vi "음료자판기.vi"() -> ()   [LabVIEW 2014]
uses:
  <vilib>/Utility/miscctls.llb/LVOutOfRangeActionTypeDef.ctl
panel:
  in  "음료선택":u8(knob) max=2 step=1 scale=0.0..2.0
  in  "정지":bool
  in  "구매":bool
  in  "음료수량 초기값":cluster{"콜라":u8, "사이다":u8, "생수":u8}={"콜라"=10, "사이다"=10, "생수"=10}
  out "생수":u8
  out "사이다":u8
  out "콜라":u8
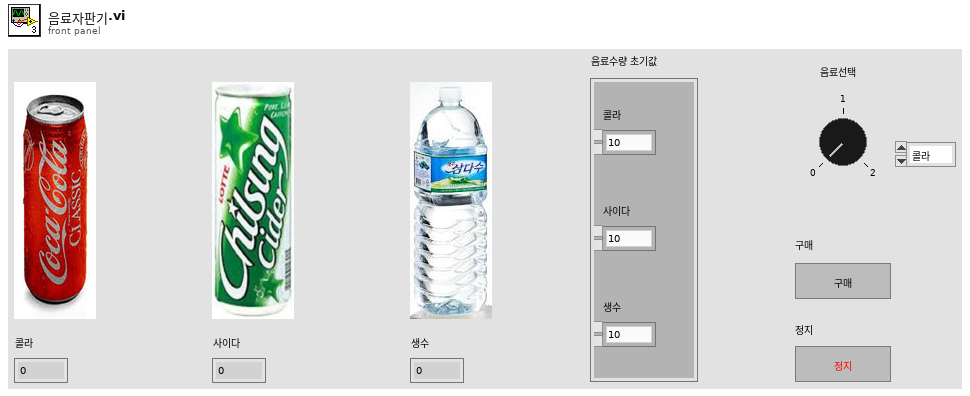
[diagram p1: front panel]
types:
  T1 = typedef "음료.ctl" = enum16{"Idle", "초기화", "정지", "음료확인", "구매"}
  T2 = typedef "LVOutOfRangeActionTypeDef.ctl" = cluster{"Out of Range Action Minimum":u8, "Out of Range Action Maximum":u8, "Out of Range Action Increment":u8}
  T3 = enum8{"Enabled", "Disabled", "Disabled and Grayed Out"}
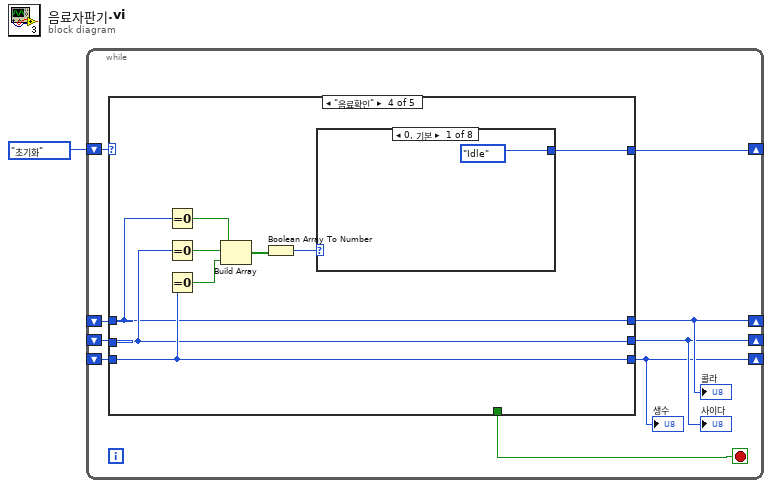
[diagram p0: block diagram]
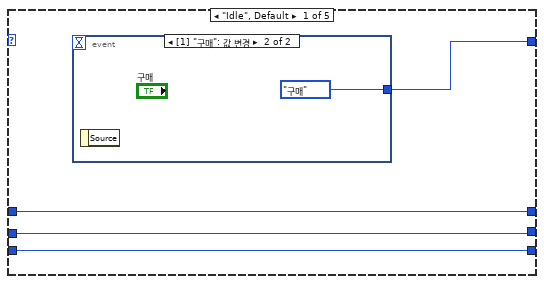
[diagram p2: hidden frame]
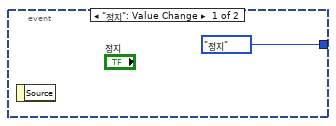
[diagram p3: hidden frame]
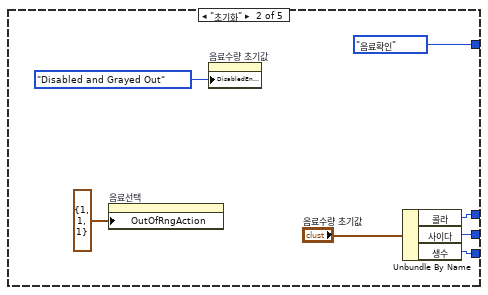
[diagram p4: hidden frame]
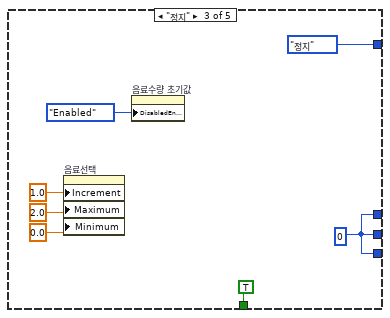
[diagram p5: hidden frame]
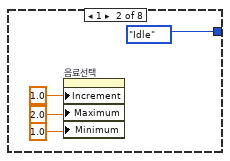
[diagram p6: hidden frame]
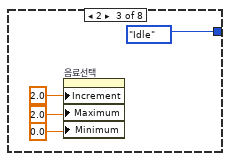
[diagram p7: hidden frame]
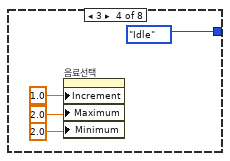
[diagram p8: hidden frame]
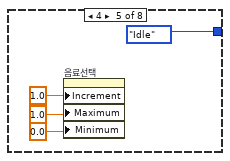
[diagram p9: hidden frame]
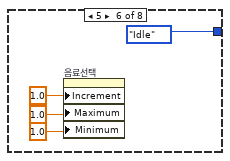
[diagram p10: hidden frame]
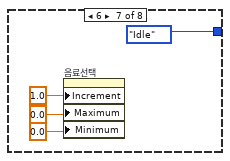
[diagram p11: hidden frame]
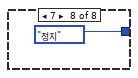
[diagram p12: hidden frame]
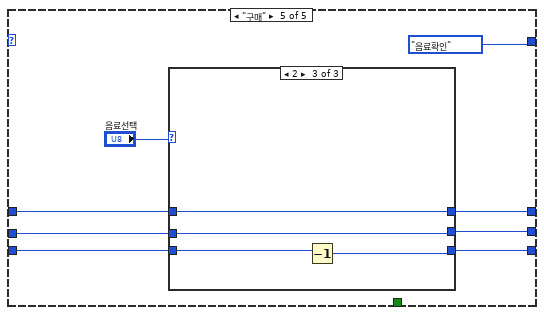
[diagram p13: hidden frame]
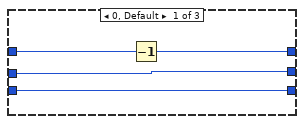
[diagram p14: hidden frame]
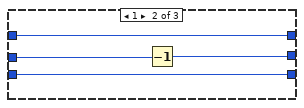
[diagram p15: hidden frame]
diagram:
  n1 = while {
    shift-right: [w9] -> _
    shift-left: 음료."초기화" ("열거형") -> [w10]
    shift-right: [w4] -> _
    shift-left: _ -> [w8]
    shift-right: [w3] -> _
    shift-left: _ -> [w7]
    shift-right: [w2] -> _
    shift-left: _ -> [w6]
    stop <- w5 stop-if-true
    n2 = case shown="\"음료확인\"" w10 {
      tunnel: [w14 음료."음료확인" ("열거형") 음료."정지" ("열거형") w31 음료."음료확인" ("열거형")] -> w9
      tunnel: w8 -> [w13 _ _ w37 w72]
      tunnel: w7 -> [w12 _ _ w38 w69]
      tunnel: w6 -> [w11 _ _ w39 w67]
      tunnel: [w13 w21 w24 w37 w71] -> w4
      tunnel: [w12 w20 w24 w38 w70] -> w3
      tunnel: [w11 w19 w24 w39 w68] -> w2
      tunnel: [_ _ TRUE _ _] -> w5
      frame "Idle", Default {
        n3 = event shown="[1] \"구매\": 값 변경" {
          selector: _ -> [_ _]
          dyn-events: _ -> [_ _]
          timeout: _ -> [_ _]
          tunnel: [음료."정지" ("열거형") 음료."구매" ("열거형")] -> w14
          event "정지": Value Change {
            n4 = event-data() -> ()  [unwired: 1 in, 1 out]
          }
          event "구매": Value Change {
            n5 = event-data() -> ()  [unwired: 1 in, 1 out]
          }
        }
      }
      frame "초기화" {
        n6 = property on="음료선택" class="Knob (엄격한)"("OutOfRngAction"=T2 {"Out of Range Action Minimum"=1, "Out of Range Action Maximum"=1, "Out of Range Action Increment"=1} ("리미트 밖의 값에 응답")) -> ()  [unwired: 2 in, 2 out]
        n7 = property on="음료수량 초기값" class="Clust (엄격한)"("DisabledEnum"=T3."Disabled and Grayed Out" ("비활성화")) -> ()  [unwired: 2 in, 2 out]
        n8 = Unbundle By Name("음료수량 초기값") -> ("콜라"=w21:u8, "사이다"=w20:u8, "생수"=w19:u8)
      }
      frame "정지" {
        w24 = 0
        n9 = property on="음료선택" class="Knob (엄격한)"("Increment"=1.0 ("데이터 입력 제한:증가"), "Maximum"=2.0 ("데이터 입력 제한:최대"), "Minimum"=0.0 ("데이터 입력 제한:최소")) -> ()  [unwired: 2 in, 2 out]
        n10 = property on="음료수량 초기값" class="Clust (엄격한)"("DisabledEnum"=T3."Enabled" ("비활성화")) -> ()  [unwired: 2 in, 2 out]
      }
      frame "음료확인" {
        n11 = Equal To 0?(x=w37) -> (x = 0?=w36:bool)
        n12 = Equal To 0?(x=w38) -> (x = 0?=w35:bool)
        n13 = Equal To 0?(x=w39) -> (x = 0?=w34:bool)
        n14 = Build Array(w36, w35, w34) -> (w33:bool[])
        n15 = Boolean Array To Number(Boolean array=w33) -> (number=w32:u32)
        n16 = case shown="0, 기본" w32 {
          tunnel: [음료."Idle" ("열거형") 음료."Idle" ("열거형") 음료."Idle" ("열거형") 음료."Idle" ("열거형") 음료."Idle" ("열거형") 음료."Idle" ("열거형") 음료."Idle" ("열거형") 음료."정지" ("열거형")] -> w31
          frame 0, Default {
          }
          frame 1 {
            n17 = property on="음료선택" class="Knob (엄격한)"("Increment"=1.0 ("데이터 입력 제한:증가"), "Maximum"=2.0 ("데이터 입력 제한:최대"), "Minimum"=1.0 ("데이터 입력 제한:최소")) -> ()  [unwired: 2 in, 2 out]
          }
          frame 2 {
            n18 = property on="음료선택" class="Knob (엄격한)"("Increment"=2.0 ("데이터 입력 제한:증가"), "Maximum"=2.0 ("데이터 입력 제한:최대"), "Minimum"=0.0 ("데이터 입력 제한:최소")) -> ()  [unwired: 2 in, 2 out]
          }
          frame 3 {
            n19 = property on="음료선택" class="Knob (엄격한)"("Increment"=1.0 ("데이터 입력 제한:증가"), "Maximum"=2.0 ("데이터 입력 제한:최대"), "Minimum"=2.0 ("데이터 입력 제한:최소")) -> ()  [unwired: 2 in, 2 out]
          }
          frame 4 {
            n20 = property on="음료선택" class="Knob (엄격한)"("Increment"=1.0 ("데이터 입력 제한:증가"), "Maximum"=1.0 ("데이터 입력 제한:최대"), "Minimum"=0.0 ("데이터 입력 제한:최소")) -> ()  [unwired: 2 in, 2 out]
          }
          frame 5 {
            n21 = property on="음료선택" class="Knob (엄격한)"("Increment"=1.0 ("데이터 입력 제한:증가"), "Maximum"=1.0 ("데이터 입력 제한:최대"), "Minimum"=1.0 ("데이터 입력 제한:최소")) -> ()  [unwired: 2 in, 2 out]
          }
          frame 6 {
            n22 = property on="음료선택" class="Knob (엄격한)"("Increment"=1.0 ("데이터 입력 제한:증가"), "Maximum"=0.0 ("데이터 입력 제한:최대"), "Minimum"=0.0 ("데이터 입력 제한:최소")) -> ()  [unwired: 2 in, 2 out]
          }
          frame 7 {
          }
        }
      }
      frame "구매" {
        n23 = case shown="2" "음료선택" {
          tunnel: w72 -> [w77 w81 w82]
          tunnel: [w76 w81 w82] -> w71
          tunnel: [w75 w79 w83] -> w70
          tunnel: w69 -> [w75 w80 w83]
          tunnel: [w74 w78 w84] -> w68
          tunnel: w67 -> [w74 w78 w85]
          frame 0, Default {
            n24 = Decrement(x=w77) -> (x-1=w76:i32)
          }
          frame 1 {
            n25 = Decrement(x=w80) -> (x-1=w79:i32)
          }
          frame 2 {
            n26 = Decrement(x=w85) -> (x-1=w84:i32)
          }
        }
      }
    }
    "콜라" <- w4
    "사이다" <- w3
    "생수" <- w2
  }
